vi "LV2G ScriptEditorSettings.vi"(7 "Operation":T2, 8 "error in (no error)":errorcluster, 11 "Script Editor Settings":T1) -> (0 "error out":errorcluster, 3 "Script Editor Settings Out":T1)   [LabVIEW 2011]
uses:
  Strict Type Controls/Settings Operation.ctl
  Strict Type Controls/ScriptEditorSettings.ctl
  <vilib>/Utility/config.llb/NI_LVConfig.lvlib
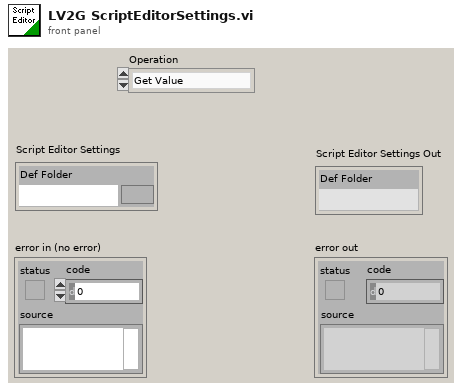
[diagram p1: front panel]
types:
  T1 = typedef "ScriptEditorSettings.ctl" = cluster{"Def Folder":path}
  T2 = typedef "Settings Operation.ctl" = enum8{"Get Value", "Set Value", "Read File", "Write File", "Write Stored Value"}
  T3 = typedef "NI_LVConfig.lvlib/Config Data RefNum.ctl" = refnum<k1>
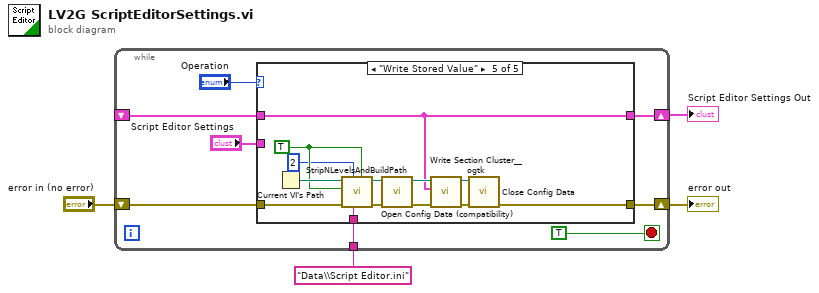
[diagram p0: block diagram]
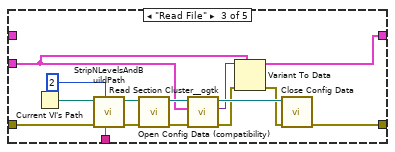
[diagram p4: hidden frame]
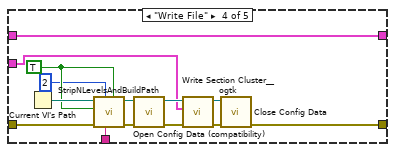
[diagram p5: hidden frame]
diagram:
  n1 = while {
    shift-right: [w8] -> w3
    shift-left: _ -> [w12]
    shift-right: [w9] -> w2
    shift-left: "error in (no error)" -> [w10]
    tunnel: "Data\\Script Editor.ini" ("string") -> [w6]
    stop <- TRUE stop-if-true
    n2 = case shown="\"Write Stored Value\"" "Operation" {
      tunnel: w12 -> [w14 _ _ w32 w50]
      tunnel: [w14 w15 w21 w32 w50] -> w8
      tunnel: "Script Editor Settings" -> [_ w15 w19 w33 _]
      tunnel: w10 -> [w13 w16 w30 w44 w57]
      tunnel: [w13 w16 w18 w36 w48] -> w9
      tunnel: w6 -> [_ _ w20 w37 w49]
      frame "Get Value" {
      }
      frame "Set Value" {
      }
      frame "Read File" {
        n3 = Current VI's Path() -> (path=w31:path)
        n4 = call "StripNLevelsAndBuildPath.vi"("Build Path"=w20, "Strip Levels"=2, "error in(no error)"=w30, "Path In"=w31) -> ("error out"=w28:errorcluster, "Path Out"=w29:path)  [unwired: 2 in, 4 out]
        n5 = call <vilib>:"Open Config Data (compatibility).vi"("error in (no error)"=w28, "configuration file path"=w29) -> ("error out"=w26:errorcluster, "refnum"=w27:T3)  [unwired: 7 in, 1 out]
        n6 = call <userlib>:"Read Section Cluster__ogtk.vi"("error in (no error)"=w26, "Section Formatted Cluster Type"=w19, "refnum"=w27) -> ("error out"=w23:errorcluster, "Section Formatted Cluster"=w24:variant, "dup refnum"=w25:T3)  [unwired: 6 out]
        n7 = Variant To Data(error in=w23, type=w19, Variant=w24) -> (data=w21:T1, error out=w22:errorcluster)
        n8 = call <vilib>:"Close Config Data.vi"("error in (no error)"=w22, "refnum"=w25) -> ("error out"=w18:errorcluster)  [unwired: 1 in, 8 out]
      }
      frame "Write File" {
        w35 = TRUE ("Create Folders")
        n9 = Current VI's Path() -> (path=w45:path)
        n10 = call "StripNLevelsAndBuildPath.vi"("Create Folders"=w35, "Build Path"=w37, "Strip Levels"=2, "error in(no error)"=w44, "Is File"=w35, "Path In"=w45) -> ("error out"=w40:errorcluster, "Path Out"=w39:path)  [unwired: 4 out]
        n11 = call <vilib>:"Open Config Data (compatibility).vi"("error in (no error)"=w40, "configuration file path"=w39) -> ("error out"=w42:errorcluster, "refnum"=w43:T3)  [unwired: 7 in, 1 out]
        n12 = call <userlib>:"Write Section Cluster__ogtk.vi"("error in (no error)"=w42, "Section Formatted Cluster"=w33, "refnum"=w43) -> ("error out"=w38:errorcluster, "dup refnum"=w41:T3)  [unwired: 1 in, 6 out]
        n13 = call <vilib>:"Close Config Data.vi"("error in (no error)"=w38, "refnum"=w41) -> ("error out"=w36:errorcluster)  [unwired: 1 in, 8 out]
      }
      frame "Write Stored Value" {
        w47 = TRUE ("Create Folders")
        n14 = Current VI's Path() -> (path=w58:path)
        n15 = call "StripNLevelsAndBuildPath.vi"("Create Folders"=w47, "Build Path"=w49, "Strip Levels"=2, "error in(no error)"=w57, "Is File"=w47, "Path In"=w58) -> ("error out"=w53:errorcluster, "Path Out"=w52:path)  [unwired: 4 out]
        n16 = call <vilib>:"Open Config Data (compatibility).vi"("error in (no error)"=w53, "configuration file path"=w52) -> ("error out"=w55:errorcluster, "refnum"=w56:T3)  [unwired: 7 in, 1 out]
        n17 = call <userlib>:"Write Section Cluster__ogtk.vi"("error in (no error)"=w55, "Section Formatted Cluster"=w50, "refnum"=w56) -> ("error out"=w51:errorcluster, "dup refnum"=w54:T3)  [unwired: 1 in, 6 out]
        n18 = call <vilib>:"Close Config Data.vi"("error in (no error)"=w51, "refnum"=w54) -> ("error out"=w48:errorcluster)  [unwired: 1 in, 8 out]
      }
    }
  }
  "error out" <- w2
  "Script Editor Settings Out" <- w3
